vi "Enqueue Message (Enum).vi"(6 "Priority Message? (F)":bool, 8 "error in (no error)":errorcluster, 9 "Message Data":variant, 10 "Demo Actions":T1, 11 "queue in":refnum<queue>) -> (0 "error out":errorcluster, 3 "queue out":refnum<queue>)   [LabVIEW 2014]
doc: "For a regular message, enqueue the message. For a priority message, enqueue it at the front of the queue."
uses:
  Typedefs/Demo Actions.ctl
  Typedefs/Message.ctl
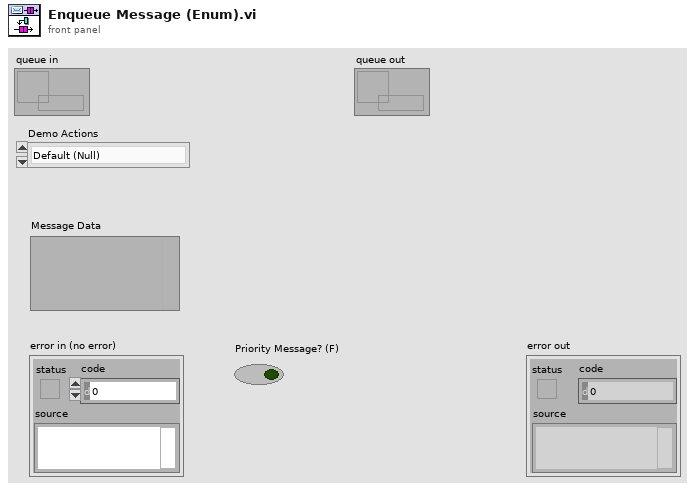
[diagram p1: front panel]
types:
  T1 = typedef "Demo Actions.ctl" = enum16{"Default (Null)", "Move (debug)", "Reset Position", "Find Home and Move to Zero", "Set Home Point", "Start", "Stop", "Pause", "Unpause"}
  T2 = typedef "Message.ctl" = cluster{"Demo Actions":T1, "Data":variant}
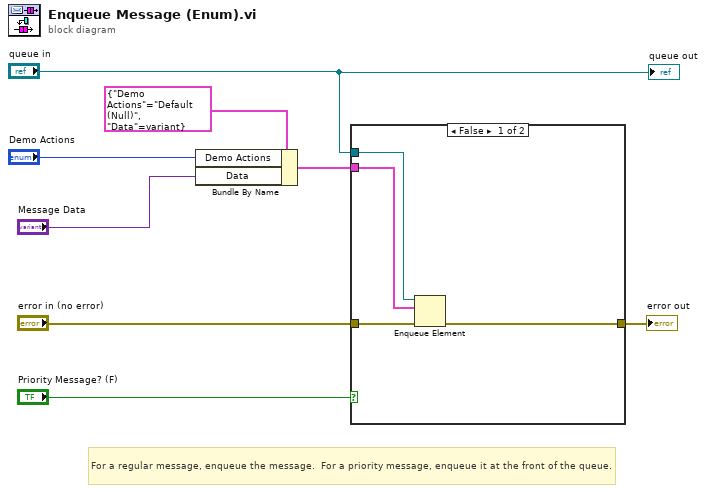
[diagram p0: block diagram]
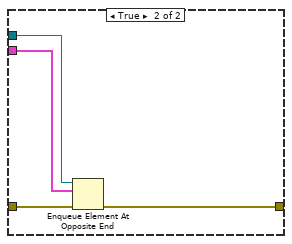
[diagram p2: hidden frame]
diagram:
  # "For a regular message, enqueue the message.  For a priority message, enqueue it at the front of the queue."
  n1 = Bundle By Name(cluster=T2 {"Demo Actions"=enum."Default (Null)", "Data"=variant} ("Message"), "Demo Actions"="Demo Actions", "Data"="Message Data") -> (w4:T2)
  n2 = case shown="False" "Priority Message? (F)" {
    tunnel: "error in (no error)" -> [w12 w16]
    tunnel: [w11 w15] -> w5
    tunnel: "queue in" -> [w10 w14]
    tunnel: w4 -> [w9 w13]
    frame False {
      n3 = Enqueue Element(queue=w10, element=w9, error in (no error)=w12) -> (error out=w11:errorcluster)  [unwired: 1 in, 2 out]
    }
    frame True {
      n4 = Enqueue Element At Opposite End(queue=w14, element=w13, error in (no error)=w16) -> (error out=w15:errorcluster)  [unwired: 1 in, 2 out]
    }
  }
  "error out" <- w5
  "queue out" <- "queue in"
